vi "Connect.vi"() -> (0 "error out":errorcluster {"code" format="%.0x"}, 2 "Connected":bool, 3 "VISA resource name out":refnum<visa-resource-name>)   [LabVIEW 2015]
doc: "Use this block at the start of an ESP301 program. It runs some stuff that came with the box that will get it all connected. There's probably a way to have it connect without pop ups and things but I dont know it.a"
uses:
  <userlib>/Newport ESP301/Newport ESP301.lvlib
panel:
  # "Use this block at the start of an ESP301 program.\nIt runs some stuff that came with the box that \nwill get it all connected. This needs to be run at \nthe beggining of any program where you want \nto communicate with the ESP 301"
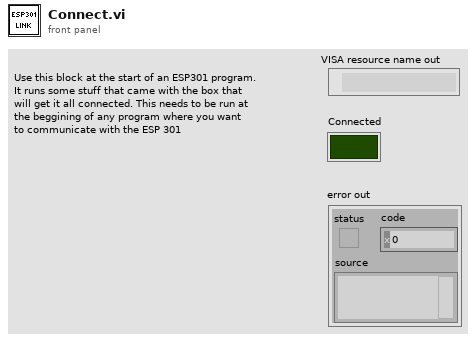
[diagram p1: front panel]
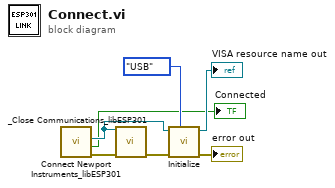
[diagram p0: block diagram]
diagram:
  n1 = call <userlib>:"Connect Newport Instruments_libESP301.vi"() -> ("error (duplicate)"=w5:errorcluster, "Connected"=→"Connected":bool, "VISA resource name (duplicate)"=w4:refnum<visa-resource-name>)  [unwired: 7 in, 2 out]
  n2 = call <userlib>:"_Close Communications_libESP301.vi"("Instrument Channel"=w4, "error in (no error)"=w5) -> ("error out"=w7:errorcluster)  [unwired: 13 in]
  n3 = call <userlib>:"Initialize.vi"("VISA resource name"=w4, "error in (no error)"=w7, "Serial Link (USB)"=enum16{"RS232", "USB"}."USB" ("Serial Link (RS232)")) -> ("VISA resource name out"=→"VISA resource name out":refnum<visa-resource-name>, "error out"=→"error out":errorcluster)  [unwired: 6 in]
